vi "Result_distance_GPS(Subvi).vi"(0 "아이템 이름":string[][](array[string])) -> (1 "1_2_distance[m]":dbl, 2 "1_3_distance[m]":dbl, 3 "1_4_distance[m]":dbl, 4 "1_5_distance[m]":dbl, 6 "2_3_distance[m]":dbl, 8 "2_4_distance[m]":dbl, 10 "2_5_distance[m]":dbl, 13 "4_5_distance[m]":dbl, 14 "3_5_distance[m]":dbl, 15 "3_4_distance[m]":dbl)   [LabVIEW 2024]
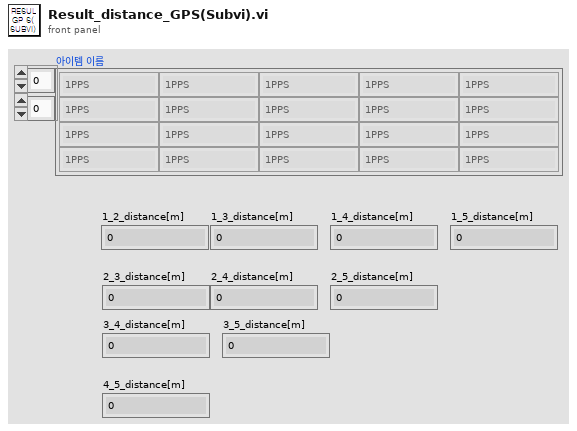
[diagram p1: front panel]
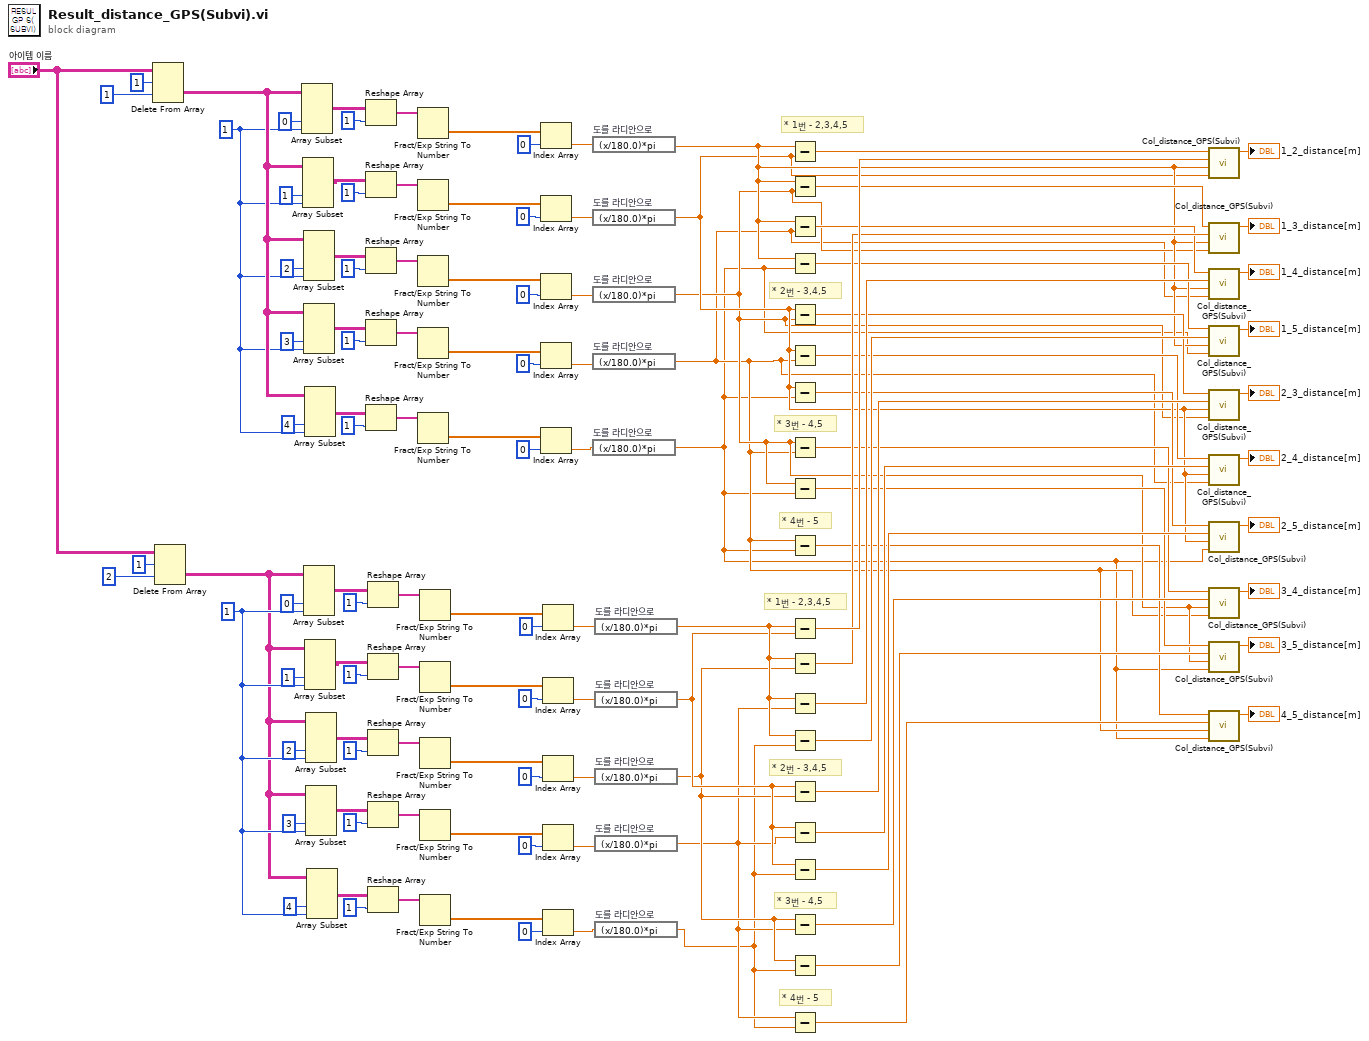
[diagram p0: block diagram]
diagram:
  w50 = 1 ("길이")
  w111 = 1 ("길이")
  # "* 4번 - 5"
  # "* 3번 - 4,5"
  # "* 2번 - 3,4,5"
  # "* 1번 - 2,3,4,5"
  # "* 4번 - 5"
  # "* 3번 - 4,5"
  # "* 2번 - 3,4,5"
  # "* 1번 - 2,3,4,5"
  n1 = Delete From Array(array="아이템 이름", length=1 ("길이"), index (row)=1 ("인덱스 (행)")) -> (deleted portion=w113:string[][])  [unwired: 1 in, 1 out]
  n2 = Delete From Array(array="아이템 이름", length=1 ("길이"), index (row)=2 ("인덱스 (행)")) -> (deleted portion=w48:string[][])  [unwired: 1 in, 1 out]
  n3 = Array Subset(array=w113, index (col)=0 ("인덱스"), length (col)=w111) -> (w108:string[][])  [unwired: 2 in]
  n4 = Array Subset(array=w113, index (col)=1 ("인덱스"), length (col)=w111) -> (w105:string[][])  [unwired: 2 in]
  n5 = Array Subset(array=w113, index (col)=2 ("인덱스"), length (col)=w111) -> (w98:string[][])  [unwired: 2 in]
  n6 = Array Subset(array=w113, index (col)=3 ("인덱스"), length (col)=w111) -> (w97:string[][])  [unwired: 2 in]
  n7 = Array Subset(array=w48, index (col)=0 ("인덱스"), length (col)=w50) -> (w53:string[][])  [unwired: 2 in]
  n8 = Array Subset(array=w113, index (col)=4 ("인덱스"), length (col)=w111) -> (w96:string[][])  [unwired: 2 in]
  n9 = Array Subset(array=w48, index (col)=1 ("인덱스"), length (col)=w50) -> (w56:string[][])  [unwired: 2 in]
  n10 = Array Subset(array=w48, index (col)=2 ("인덱스"), length (col)=w50) -> (w63:string[][])  [unwired: 2 in]
  n11 = Array Subset(array=w48, index (col)=3 ("인덱스"), length (col)=w50) -> (w64:string[][])  [unwired: 2 in]
  n12 = Array Subset(array=w48, index (col)=4 ("인덱스"), length (col)=w50) -> (w65:string[][])  [unwired: 2 in]
  n13 = Reshape Array(w108, 1 ("차원 크기")) -> (w110:string[])
  n14 = Reshape Array(w105, 1 ("차원 크기")) -> (w106:string[])
  n15 = Reshape Array(w98, 1 ("차원 크기")) -> (w104:string[])
  n16 = Reshape Array(w97, 1 ("차원 크기")) -> (w101:string[])
  n17 = Reshape Array(w96, 1 ("차원 크기")) -> (w100:string[])
  n18 = Reshape Array(w53, 1 ("차원 크기")) -> (w51:string[])
  n19 = Reshape Array(w56, 1 ("차원 크기")) -> (w55:string[])
  n20 = Reshape Array(w63, 1 ("차원 크기")) -> (w57:string[])
  n21 = Reshape Array(w64, 1 ("차원 크기")) -> (w60:string[])
  n22 = Reshape Array(w65, 1 ("차원 크기")) -> (w61:string[])
  n23 = Fract/Exp String To Number(string=w110) -> (number=w94:dbl[])  [unwired: 3 in, 1 out]
  n24 = Fract/Exp String To Number(string=w106) -> (number=w92:dbl[])  [unwired: 3 in, 1 out]
  n25 = Fract/Exp String To Number(string=w104) -> (number=w88:dbl[])  [unwired: 3 in, 1 out]
  n26 = Fract/Exp String To Number(string=w101) -> (number=w87:dbl[])  [unwired: 3 in, 1 out]
  n27 = Fract/Exp String To Number(string=w100) -> (number=w86:dbl[])  [unwired: 3 in, 1 out]
  n28 = Fract/Exp String To Number(string=w51) -> (number=w67:dbl[])  [unwired: 3 in, 1 out]
  n29 = Fract/Exp String To Number(string=w55) -> (number=w69:dbl[])  [unwired: 3 in, 1 out]
  n30 = Fract/Exp String To Number(string=w57) -> (number=w73:dbl[])  [unwired: 3 in, 1 out]
  n31 = Fract/Exp String To Number(string=w60) -> (number=w74:dbl[])  [unwired: 3 in, 1 out]
  n32 = Fract/Exp String To Number(string=w61) -> (number=w75:dbl[])  [unwired: 3 in, 1 out]
  n33 = Index Array(array=w94, index=0 ("인덱스")) -> (element=w85:dbl)
  n34 = Index Array(array=w92, index=0 ("인덱스")) -> (element=w84:dbl)
  n35 = Index Array(array=w88, index=0 ("인덱스")) -> (element=w83:dbl)
  n36 = Index Array(array=w87, index=0 ("인덱스")) -> (element=w82:dbl)
  n37 = Index Array(array=w86, index=0 ("인덱스")) -> (element=w81:dbl)
  n38 = Index Array(array=w67, index=0 ("인덱스")) -> (element=w76:dbl)
  n39 = Index Array(array=w69, index=0 ("인덱스")) -> (element=w77:dbl)
  n40 = Index Array(array=w73, index=0 ("인덱스")) -> (element=w78:dbl)
  n41 = Index Array(array=w74, index=0 ("인덱스")) -> (element=w79:dbl)
  n42 = Index Array(array=w75, index=0 ("인덱스")) -> (element=w80:dbl)
  n43 = expression code="(x/180.0)*pi" "도를 라디안으로"(w85) -> (w5:dbl)
  n44 = expression code="(x/180.0)*pi" "도를 라디안으로"(w84) -> (w4:dbl)
  n45 = expression code="(x/180.0)*pi" "도를 라디안으로"(w83) -> (w3:dbl)
  n46 = expression code="(x/180.0)*pi" "도를 라디안으로"(w82) -> (w2:dbl)
  n47 = expression code="(x/180.0)*pi" "도를 라디안으로"(w81) -> (w1:dbl)
  n48 = expression code="(x/180.0)*pi" "도를 라디안으로"(w76) -> (w40:dbl)
  n49 = expression code="(x/180.0)*pi" "도를 라디안으로"(w77) -> (w39:dbl)
  n50 = expression code="(x/180.0)*pi" "도를 라디안으로"(w78) -> (w38:dbl)
  n51 = expression code="(x/180.0)*pi" "도를 라디안으로"(w79) -> (w37:dbl)
  n52 = expression code="(x/180.0)*pi" "도를 라디안으로"(w80) -> (w36:dbl)
  n53 = Subtract(x=w5, y=w4) -> (x-y=w35:dbl)
  n54 = Subtract(x=w5, y=w3) -> (x-y=w32:dbl)
  n55 = Subtract(x=w5, y=w2) -> (x-y=w29:dbl)
  n56 = Subtract(x=w5, y=w1) -> (x-y=w26:dbl)
  n57 = Subtract(x=w4, y=w3) -> (x-y=w23:dbl)
  n58 = Subtract(x=w4, y=w2) -> (x-y=w20:dbl)
  n59 = Subtract(x=w4, y=w1) -> (x-y=w17:dbl)
  n60 = Subtract(x=w3, y=w2) -> (x-y=w14:dbl)
  n61 = Subtract(x=w3, y=w1) -> (x-y=w11:dbl)
  n62 = Subtract(x=w2, y=w1) -> (x-y=w8:dbl)
  n63 = Subtract(x=w40, y=w39) -> (x-y=w34:dbl)
  n64 = Subtract(x=w40, y=w38) -> (x-y=w31:dbl)
  n65 = Subtract(x=w40, y=w37) -> (x-y=w28:dbl)
  n66 = Subtract(x=w40, y=w36) -> (x-y=w25:dbl)
  n67 = Subtract(x=w39, y=w38) -> (x-y=w22:dbl)
  n68 = Subtract(x=w39, y=w37) -> (x-y=w19:dbl)
  n69 = Subtract(x=w39, y=w36) -> (x-y=w16:dbl)
  n70 = Subtract(x=w38, y=w37) -> (x-y=w13:dbl)
  n71 = Subtract(x=w38, y=w36) -> (x-y=w10:dbl)
  n72 = Subtract(x=w37, y=w36) -> (x-y=w7:dbl)
  n73 = call "Col_distance_GPS(Subvi).vi"("2_위도"=w4, "1_위도"=w5, "Delta_lon"=w34, "Delta_lat"=w35) -> ("distance[m]"=→"1_2_distance[m]":dbl)  [unwired: 7 in]
  n74 = call "Col_distance_GPS(Subvi).vi"("2_위도"=w3, "1_위도"=w5, "Delta_lon"=w31, "Delta_lat"=w32) -> ("distance[m]"=→"1_3_distance[m]":dbl)  [unwired: 7 in]
  n75 = call "Col_distance_GPS(Subvi).vi"("2_위도"=w2, "1_위도"=w5, "Delta_lon"=w28, "Delta_lat"=w29) -> ("distance[m]"=→"1_4_distance[m]":dbl)  [unwired: 7 in]
  n76 = call "Col_distance_GPS(Subvi).vi"("2_위도"=w1, "1_위도"=w5, "Delta_lon"=w25, "Delta_lat"=w26) -> ("distance[m]"=→"1_5_distance[m]":dbl)  [unwired: 7 in]
  n77 = call "Col_distance_GPS(Subvi).vi"("2_위도"=w3, "1_위도"=w4, "Delta_lon"=w22, "Delta_lat"=w23) -> ("distance[m]"=→"2_3_distance[m]":dbl)  [unwired: 7 in]
  n78 = call "Col_distance_GPS(Subvi).vi"("2_위도"=w2, "1_위도"=w4, "Delta_lon"=w19, "Delta_lat"=w20) -> ("distance[m]"=→"2_4_distance[m]":dbl)  [unwired: 7 in]
  n79 = call "Col_distance_GPS(Subvi).vi"("2_위도"=w1, "1_위도"=w4, "Delta_lon"=w16, "Delta_lat"=w17) -> ("distance[m]"=→"2_5_distance[m]":dbl)  [unwired: 7 in]
  n80 = call "Col_distance_GPS(Subvi).vi"("2_위도"=w2, "1_위도"=w3, "Delta_lon"=w13, "Delta_lat"=w14) -> ("distance[m]"=→"3_4_distance[m]":dbl)  [unwired: 7 in]
  n81 = call "Col_distance_GPS(Subvi).vi"("2_위도"=w1, "1_위도"=w3, "Delta_lon"=w10, "Delta_lat"=w11) -> ("distance[m]"=→"3_5_distance[m]":dbl)  [unwired: 7 in]
  n82 = call "Col_distance_GPS(Subvi).vi"("2_위도"=w1, "1_위도"=w2, "Delta_lon"=w7, "Delta_lat"=w8) -> ("distance[m]"=→"4_5_distance[m]":dbl)  [unwired: 7 in]
